vi "Convert plane.vi"(4 "z step size":i32, 5 "z start position":i32, 6 "basepath name":string, 7 "File Handle":u32, 8 "error in (no error)":errorcluster, 9 "Frame Index":i32=-1, 10 "file in":path, 11 "Image in":T1) -> (0 "error out":errorcluster, 3 "Image out":T1)   [LabVIEW 2012]
uses:
  <vilib>/vision/Image Controls.llb/IMAQ Image.ctl
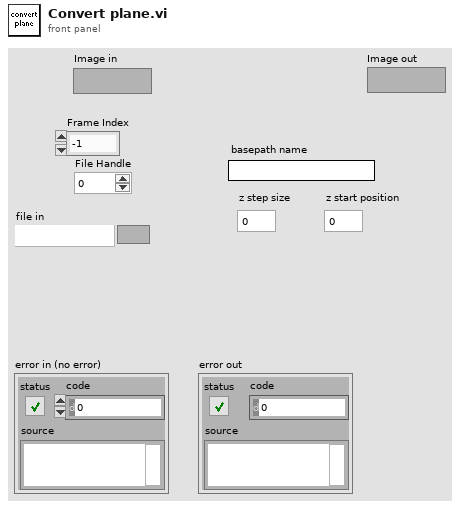
[diagram p1: front panel]
types:
  T1 = typedef "IMAQ Image.ctl" = refnum<image>
  T2 = cluster{"Rows Per Strip":i32, "Photometric":i32, "Compression Type":i32}
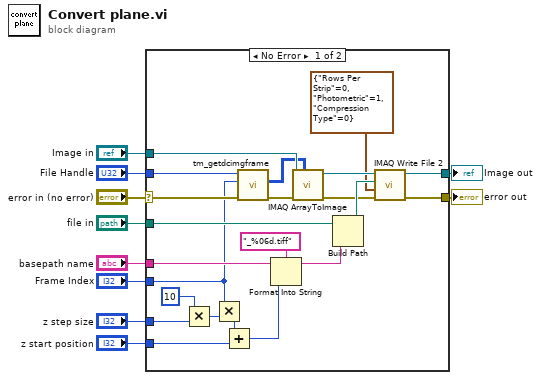
[diagram p0: block diagram]
diagram:
  n1 = case shown="No Error" "error in (no error)" {
    selector: "error in (no error)" -> [w30 w34]
    tunnel: "File Handle" -> [w32 _]
    tunnel: "file in" -> [w24 _]
    tunnel: [w28 w34] -> w8
    tunnel: "Frame Index" -> [w17 _]
    tunnel: "Image in" -> [w29 w33]
    tunnel: [w27 w33] -> w5
    tunnel: "basepath name" -> [w18 _]
    tunnel: "z step size" -> [w12 _]
    tunnel: "z start position" -> [w15 _]
    frame No Error {
      n2 = Multiply(x=10 ("y"), y=w12) -> (x*y=w11:i32)
      n3 = Multiply(x=w17, y=w11) -> (x*y=w16:i32)
      n4 = Add(x=w16, y=w15) -> (x+y=w14:i32)
      n5 = call <userlib>:"tm_getdcimgframe.vi"("error in (no error)"=w30, "Frame Index"=w17, "File Handle in"=w32) -> ("error out"=w21:errorcluster, "Data"=w22:u16[][])  [unwired: 5 in, 2 out]
      n6 = Format Into String(format string="_%06d.tiff", initial string=w18, w14) -> (resulting string=w25:string)  [unwired: 1 in, 1 out]
      n7 = call "IMAQ ArrayToImage"("Image Pixels (U16)"=w22, "error in (no error)"=w21, "Image"=w29) -> ("error out"=w20:errorcluster, "Image Out"=w23:T1)  [unwired: 7 in]
      n8 = Build Path(base path=w24, name or relative path=w25) -> (appended path=w31:path)
      n9 = call-poly "IMAQ Write File 2"("error in (no error)"=w20, "TIFF Options"=T2 {"Rows Per Strip"=0, "Photometric"=1, "Compression Type"=0}, "File Path"=w31, "Image"=w23) -> ("error out"=w28:errorcluster, "Image Out (duplicate)"=w27:T1)  [unwired: 6 in]
    }
    frame Error {
    }
  }
  "error out" <- w8
  "Image out" <- w5
